vi "Predip.vi"() -> ()   [LabVIEW 2019]
uses:
  <vilib>/NI/Current Value Table/Type Defs/Single Tag.ctl
  <vilib>/NI/Current Value Table/Type Defs/Data Types.ctl
  <vilib>/NI/STM/TCP/Read Meta Data (TCP Ref).vi
  <vilib>/NI/STM/TCP/Get Connection Reference (TCP).vi
  <vilib>/NI/AMC/Read Termination Message.vi
  <vilib>/NI/AMC/Create Single Message.vi
  <vilib>/NI/AMC/Update Message Routing Info.vi
  <vilib>/NI/STM/TCP/Read Meta Data (TCP Clst).vi
  <vilib>/NI/AMC/Globals.vi
  <vilib>/NI/STM/TCP/Write Message (TCP).vi
  <vilib>/NI/AMC/Send Message.vi
  <vilib>/NI/AMC/AMC.lvlib
  <vilib>/NI/STM/NI STM.lvlib
  <vilib>/NI/Current Value Table/Current Value Table.lvlib
panel:
  in  "Sulfuric Proc 1":dbl=2.0 caption="ml Acid Predip" min=0.0 max=2500.0 step=1.0
  in  "Trig Sulfuric Predip":bool caption="Trigger Dose"
  in  "Level Setpoint":dbl(knob)=40.0 min=40.0 max=85.0 step=0.5 scale=40.0..85.0
  in  "Enable Auto Fill":bool
  in  "AcidT3 Flow Last Hr":bool
  in  "AcidT3 Cond Last Hr":bool
  in  "AcidT3 Lev Last Hr":bool
  in  "AcidT3 T Last Hr":bool
  in  "Temperature Setpoint":dbl(knob)=25.0 min=20.0 max=55.0 step=0.5 scale=20.0..55.0
  in  "Enable Heat":bool
  out "Heater 2":bool
  out "Boolean 4":bool
  out "Boolean 2":bool
  out "Boolean 5":bool
  out "Drain":bool
  out "SuckPipe 2":bool
  out "Main Pump":bool
  in  "Tab Control":enum32{"Page 1", "ENG"}(tab)
  out "Heater Enabled":bool
  out "Amps":dbl format="%#.2g"
  out "Volts":dbl format="%#.1f"
  out "VFD T":dbl format="%#.2g"
  out "RPM":dbl format="%#.0f"
  out "Fault Code":dbl format="%#.2g"
  out "Freq":dbl format="%#.2g"
  in  "Drain Predip":bool
  out "Level (L)":dbl(slide) scale=0.0..100.0
  in  "Specific Gravity":dbl(knob)=1.0 min=1.0 max=1.3 step=0.0025 scale=1.0..1.3
  out "E Stop":bool
  out "Run Enabled?":bool
  out "Acid Temperature":dbl(slide) scale=0.0..60.0
  in  "Conductivity":dbl(slide) scale=0.1..1000.0
  in  "Flow Setpoint":dbl(knob)=25.0 min=25.0 max=100.0 step=1.0 scale=25.0..100.0
  in  "Enable Predip":bool
  out "Flow rate":dbl(knob) scale=0.0..100.0
  in  "Machine":bool
  in  "Basement 4":bool
  in  "Dryer":bool
  in  "Rinse 4":bool
  in  "Rinse 3":bool
  in  "Rinse 2":bool
  in  "Basement 3":bool
  in  "Basement 2":bool
  in  "Basement 1":bool
  in  "Plater 6":bool
  in  "Plater 5":bool
  in  "Plater 4":bool
  in  "Plater 3":bool
  in  "Plater 2":bool
  in  "Plater 1":bool
  in  "Predip":bool
  in  "Rinse 1":bool
  in  "Cleaner":bool
  in  "Etch":bool
  out "status":string
  # "Module Selection"
  # "L/min"
  # "mS"
  # "Dosing"
  # "Sulfuric Acid"
  # "Motor Parameters"
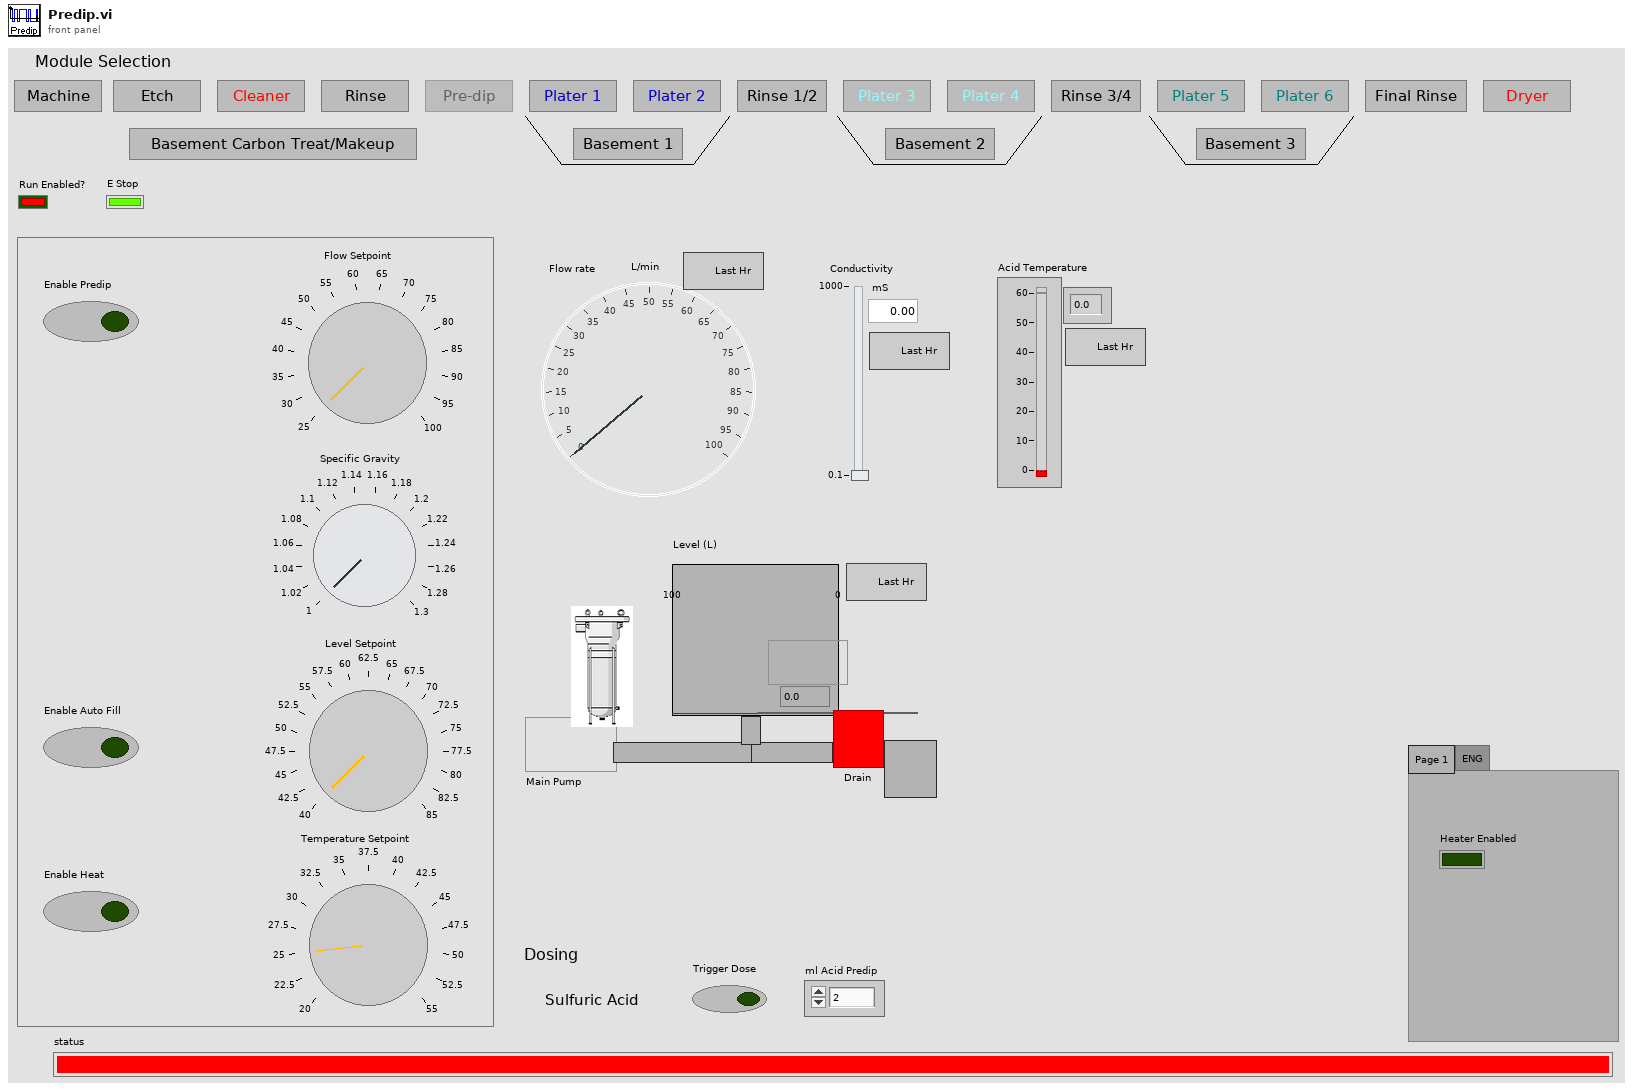
[diagram p1: front panel]
types:
  T1 = typedef "Current Value Table.lvlib/Single Tag.ctl" = cluster{"Data Type":T2, "Name":string, "Value":string, "Description":string}
  T2 = typedef "Current Value Table.lvlib/Data Types.ctl" = enum16{"Double", "Single", "I64", "I32", "I16", "I8", "U64", "U32", "U16", "U8", "String", "Boolean", "Array of U8", "Array of U16", "Array of U32", "Array of U64", "Array of I64", "Array of I32", "Array of I16", "Array of I8", "Array of Double", "Array of Single", "Array of Boolean", "Array of String"}
  T3 = typedef "NI STM.lvlib/TCP Connection Info.ctl" = cluster{"connection ID":refnum<k5>, "meta data":T4[]}
  T4 = typedef "NI STM.lvlib/MetaDataElement.ctl" = string
  T5 = typedef "AMC.lvlib/Message Queue.ctl" = refnum<queue>
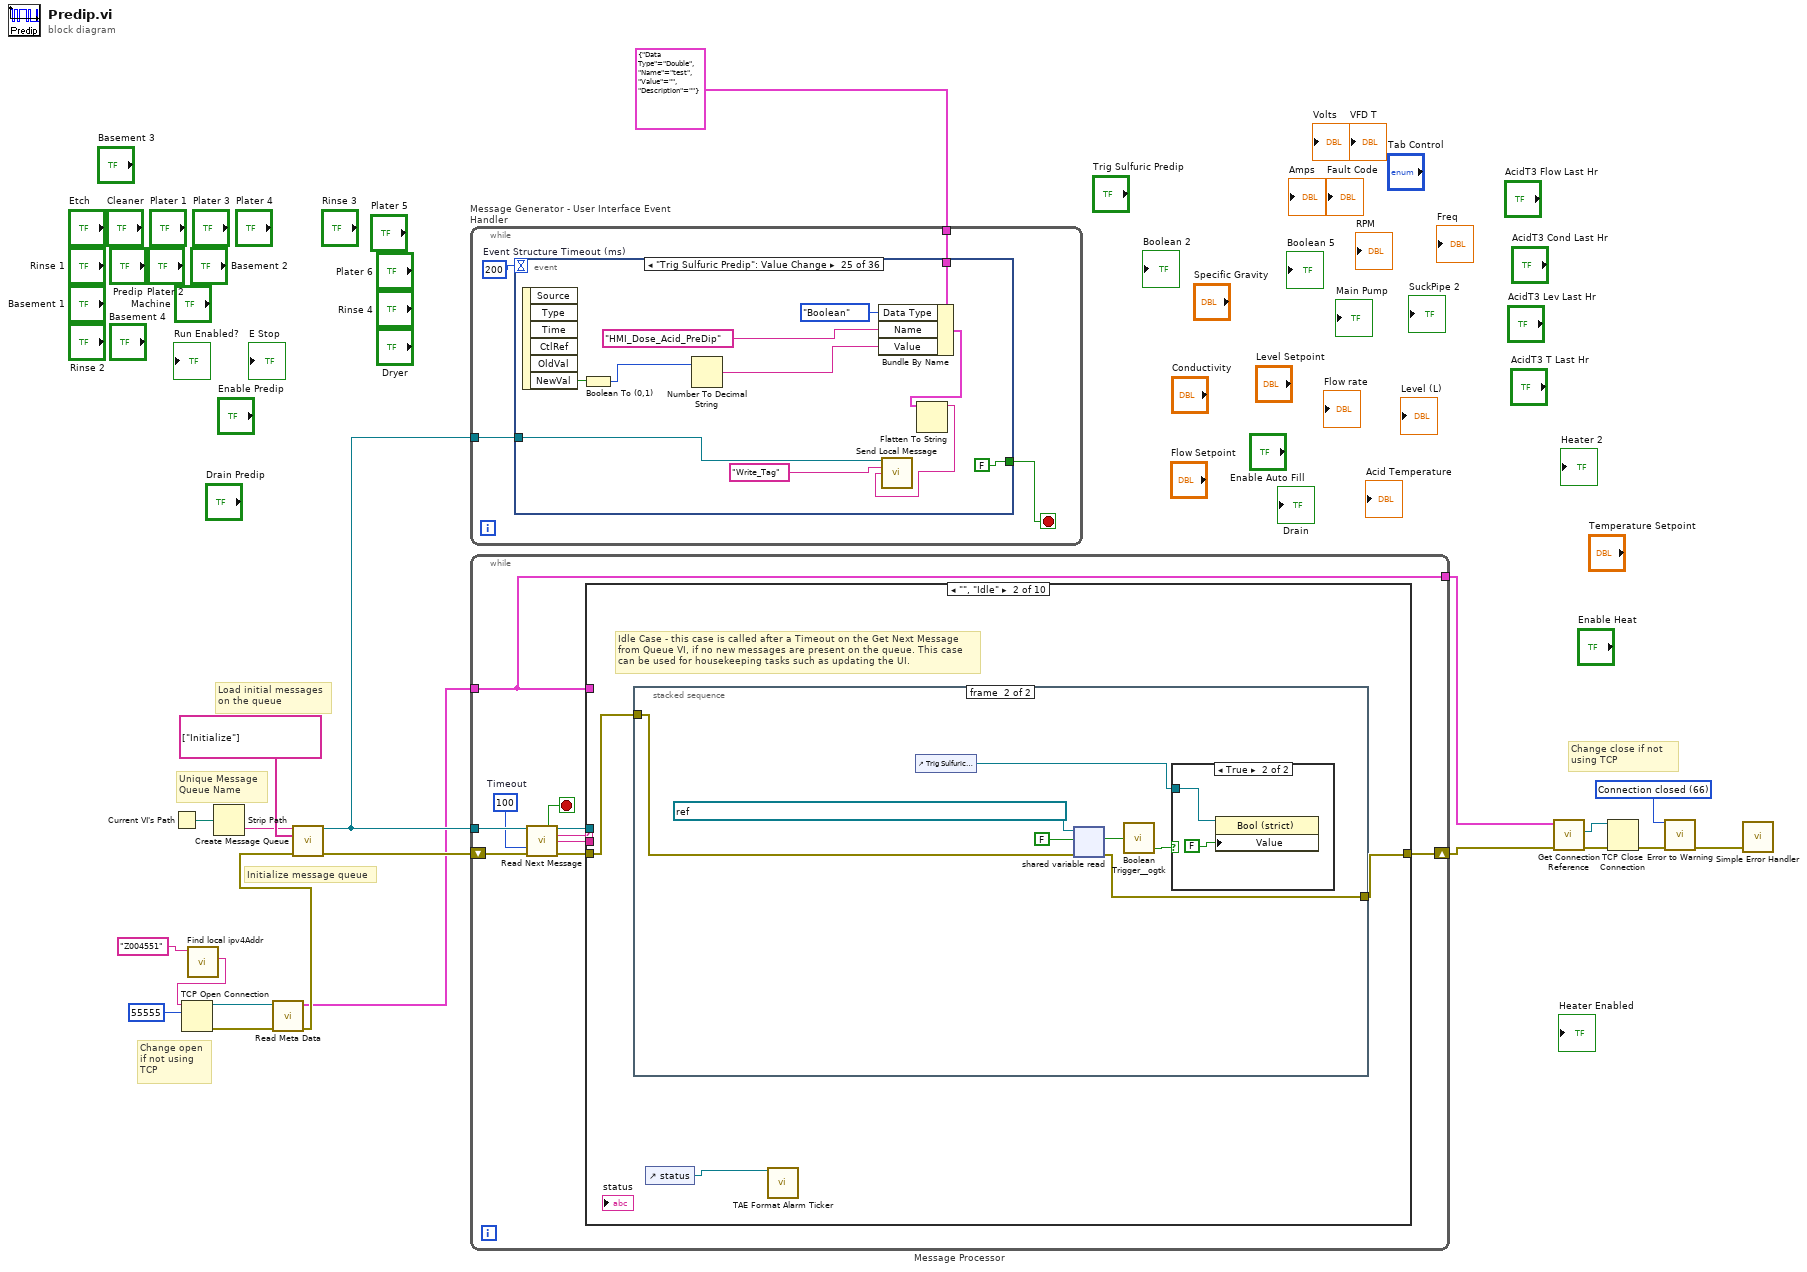
[diagram p0: block diagram]
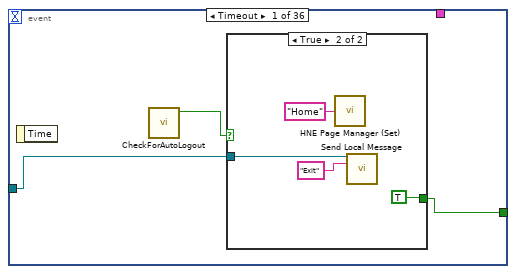
[diagram p2: hidden frame]
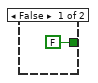
[diagram p3: hidden frame]
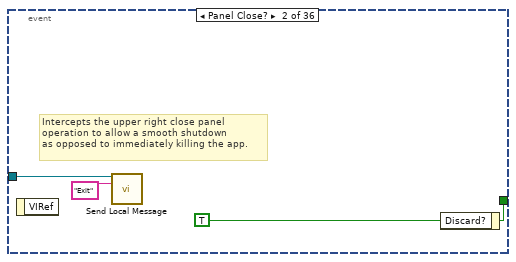
[diagram p4: hidden frame]
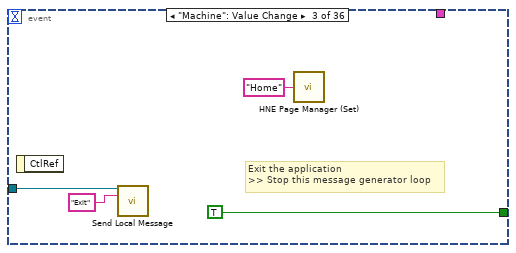
[diagram p5: hidden frame]
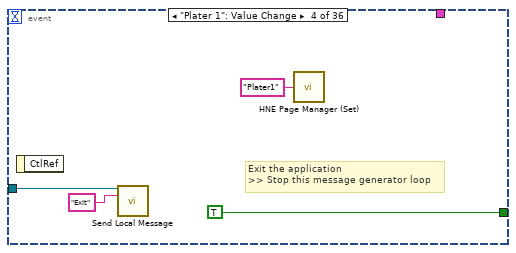
[diagram p6: hidden frame]
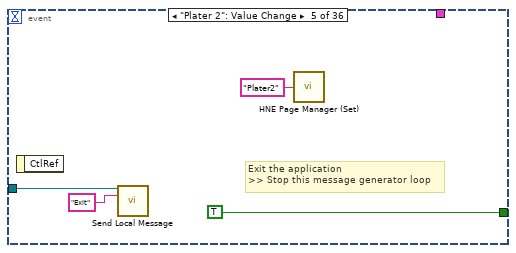
[diagram p7: hidden frame]
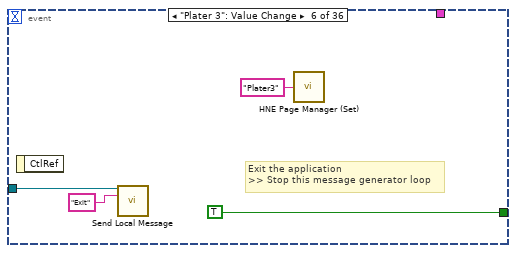
[diagram p8: hidden frame]
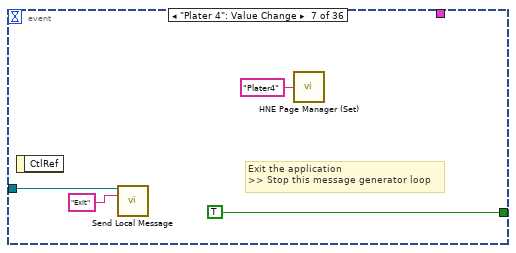
[diagram p9: hidden frame]
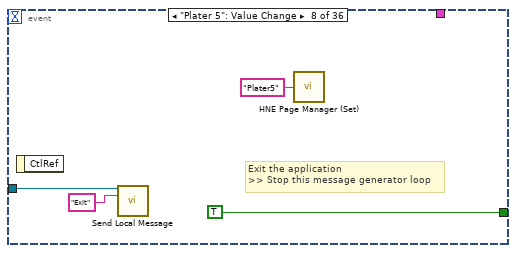
[diagram p10: hidden frame]
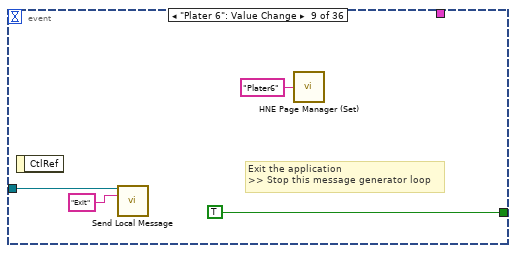
[diagram p11: hidden frame]
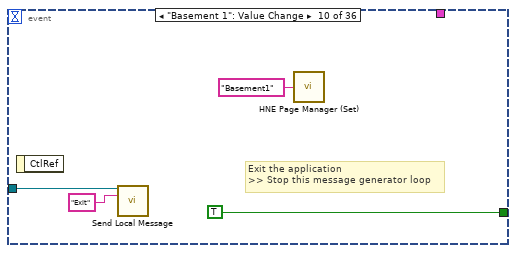
[diagram p12: hidden frame]
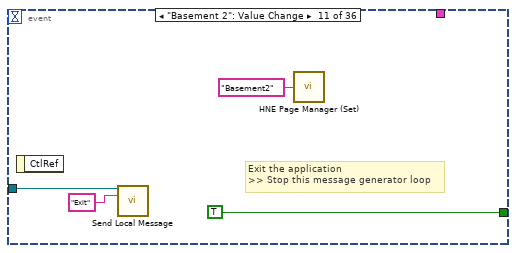
[diagram p13: hidden frame]
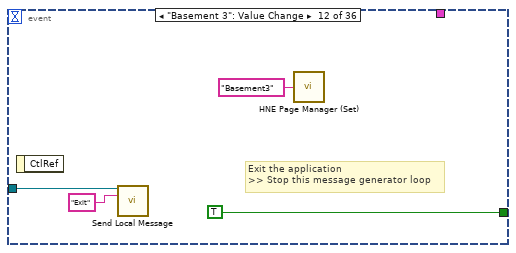
[diagram p14: hidden frame]
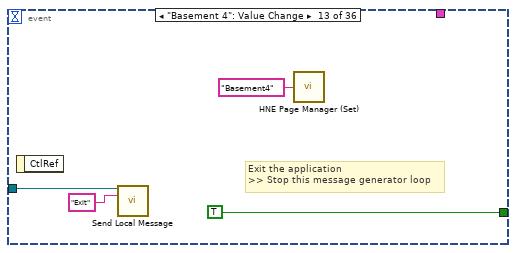
[diagram p15: hidden frame]
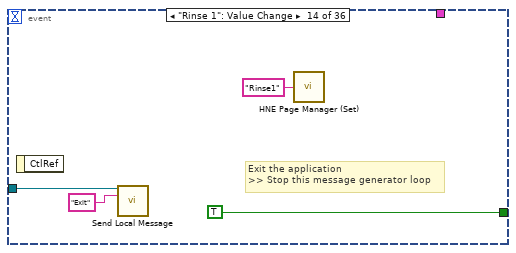
[diagram p16: hidden frame]
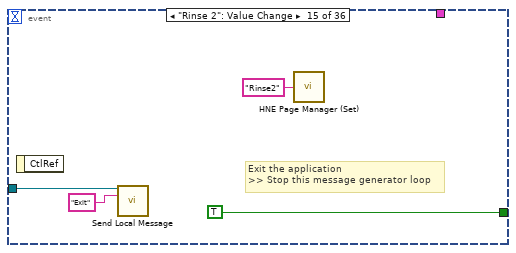
[diagram p17: hidden frame]
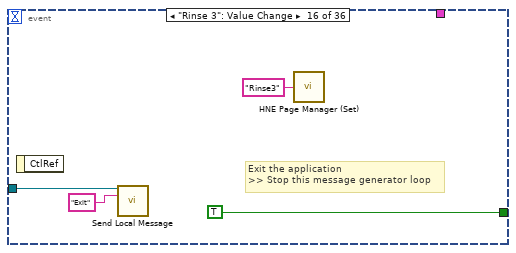
[diagram p18: hidden frame]
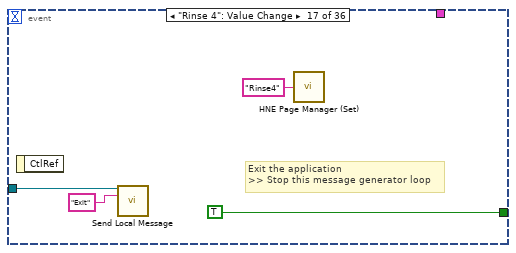
[diagram p19: hidden frame]
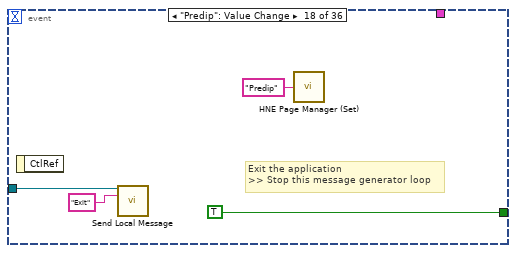
[diagram p20: hidden frame]
diagram:
  w9 = 66 items=["No Error", "Argument Error", "Memory Full", "Out of Zone", "End of File", "File Already Open", "Generic File IO Error", "File Not Found", "File Permission Error", "Disk Full", "Duplicate Path", "Too Many Files Open", "Not Enabled", "Resource File Not Found", "Cannot Add Resource", "Resource Not Found", "Image Not Found", "Image Memory Error", "Pen Does Not Exist", "Config Bad Type", "Config Token Not Found", "Config Parse Error", "Config Memory Error", "Bad External Code Format", "Bad External Code Offset", "External Code Not Present", "Null Window", "Destroy Window Mixup", "Null Menu", "Print Aborted", "Bad Print Record", "Print Driver Error", "Windows Error During Print", "Memory Error During Print", "Print Dialog Error", "Generic Print Error", "Invalid Device Refnum", "Device Not Found", "Device Parameter Error", "Device Unit Error", "Can't Open Device", "Device Call Aborted", "Generic Error", "Cancelled By User", "Object ID Too Low", "Object ID Too High", "Object Not In Heap", "Unknown Heap", "Bad DefProc ID", "DefProc Not In Table", "Message Out Of Range", "Null Method", "Unknown Message", "Manager Call Not Supported", "Bad address", "Connection In progress", "Connection timed out", "Connection is already in progress", "Network attribute not supported", "Network error", "Address in use", "System out of memory", "Connection aborted", "Connection refused", "Connection is not connected", "Connection is already connected", "Connection closed", "Initialize error (interapplication manager)", "Bad occurrence", "Wait on unbound occurrence handler", "Occurrence queue overflow", "Bad path", "Semaphore not signaled", "Unrecognized type (interapplication manager)"] ("1st Error to Convert")
  # "Change close if not using TCP"
  # "Change open if not using TCP"
  # "Initialize message queue"
  # "Unique Message\nQueue Name"
  # "Load initial messages\non the queue"
  n1 = Current VI's Path() -> (path=w16:path)
  n2 = call "Find local ipv4Addr.vi"("MachineToFind"="Z004551" ("Target IP Address")) -> ("name"=w2:string)  [unwired: 9 in, 1 out]
  n3 = TCP Open Connection(address=w2, remote port or service name=u16 55555 ("remote port")) -> (connection ID=w14:refnum<k5>, error out=w13:errorcluster)  [unwired: 1 in, 2 out]
  n4 = Strip Path(path=w16) -> (name=w19:string)  [unwired: 1 out]
  n5 = call-poly <vilib>:"Read Meta Data.vi"("error in"=w13, "connection ID"=w14) -> ("error out"=w12:errorcluster, "connection info out"=w11:T3)  [unwired: 7 in, 1 out]
  n6 = call <vilib>:"Create Message Queue.vi"("message queue name"=w19, "initial message names"=string[] ["Initialize"], "error in"=w12) -> ("message queue out"=w18:T5, "error out"=w17:errorcluster)  [unwired: 11 in]
  n7 = while "Message Generator - User Interface Event Handler" {
    tunnel: w18 -> [w22]
    tunnel: T1 {"Data Type"=enum."Double", "Name"="test", "Value"="", "Description"=""} ("Tag") -> [w21]
    stop <- w23 stop-if-true
    w24 = 200  # Event Structure Timeout (ms)
    n8 = event shown="[24] \"Trig Sulfuric Predip\": Value Change" {
      selector: _ -> [_ _ _ _ _ _ _ _ _ _ _ _ _ _ _ _ _ _ _ _ _ _ _ _ _ _ _ _ _ _ _ _ _ _ _ _]
      dyn-events: _ -> [_ _ _ _ _ _ _ _ _ _ _ _ _ _ _ _ _ _ _ _ _ _ _ _ _ _ _ _ _ _ _ _ _ _ _ _]
      timeout: w24 -> [_ _ _ _ _ _ _ _ _ _ _ _ _ _ _ _ _ _ _ _ _ _ _ _ _ _ _ _ _ _ _ _ _ _ _ _]
      tunnel: [w25 w35 TRUE ("Discard?") TRUE ("Discard?") TRUE ("Discard?") TRUE ("Discard?") TRUE ("Discard?") TRUE ("Discard?") TRUE ("Discard?") TRUE ("Discard?") TRUE ("Discard?") TRUE ("Discard?") TRUE ("Discard?") TRUE ("Discard?") TRUE ("Discard?") TRUE ("Discard?") TRUE ("Discard?") TRUE ("Discard?") TRUE ("Discard?") TRUE ("Discard?") TRUE ("Discard?") FALSE ("Discard?") FALSE ("Discard?") FALSE ("Discard?") FALSE ("Discard?") _ _ _ _ FALSE ("Discard?") FALSE ("Discard?") FALSE ("Discard?") FALSE ("Discard?") FALSE ("Discard?") FALSE ("Discard?") _] -> w23
      tunnel: w22 -> [w26 w33 w37 w41 w45 w49 w53 w57 w61 w65 w69 w73 w77 w81 w85 w89 w93 w97 w101 w105 w109 w120 w131 w142 w153 w156 w161 w166 w171 w179 w190 w200 w210 w220 w230 w233]
      tunnel: w21 -> [_ _ _ _ _ _ _ _ _ _ _ _ _ _ _ _ _ _ _ _ _ w114 w125 w136 w147 _ _ _ _ _ w186 w196 w206 w216 w226 _]
      event Timeout {
        n9 = event-data() -> ()  [unwired: 2 out]
        n10 = call "CheckForAutoLogout.vi"() -> ("Boolean"=w27:bool)  [unwired: 11 in]
        n11 = case shown="True" w27 {
          tunnel: [FALSE ("Discard?") TRUE ("Discard?")] -> w25
          tunnel: w26 -> [_ w29]
          frame False {
          }
          frame True {
            n12 = call <userlib>:"HNE Page Manager (Set).vi"("Next Page"="Home") -> ()  [unwired: 4 in, 1 out]
            n13 = call <vilib>:"Send Local Message.vi"("message queue in"=w29, "message name"="Exit") -> ()  [unwired: 11 in, 3 out]
          }
        }
      }
      event Panel Close? {
        w35 = TRUE ("Discard?")
        # "Intercepts the upper right close panel\noperation to allow a smooth shutdown\nas opposed to immediately killing the app."
        n14 = event-data() -> ()  [unwired: 2 out]
        n15 = call <vilib>:"Send Local Message.vi"("message queue in"=w33, "message name"="Exit") -> ()  [unwired: 11 in, 3 out]
        n16 = event-data("Discard?"=w35) -> ()  [unwired: 1 in, 1 out]
      }
      event "Machine": Value Change {
        # "Exit the application\n>> Stop this message generator loop"
        n17 = event-data() -> ()  [unwired: 2 out]
        n18 = call <vilib>:"Send Local Message.vi"("message queue in"=w37, "message name"="Exit") -> ()  [unwired: 11 in, 3 out]
        n19 = call <userlib>:"HNE Page Manager (Set).vi"("Next Page"="Home") -> ()  [unwired: 4 in, 1 out]
      }
      event "Plater 1": Value Change {
        # "Exit the application\n>> Stop this message generator loop"
        n20 = event-data() -> ()  [unwired: 2 out]
        n21 = call <vilib>:"Send Local Message.vi"("message queue in"=w41, "message name"="Exit") -> ()  [unwired: 11 in, 3 out]
        n22 = call <userlib>:"HNE Page Manager (Set).vi"("Next Page"="Plater1") -> ()  [unwired: 4 in, 1 out]
      }
      event "Plater 2": Value Change {
        # "Exit the application\n>> Stop this message generator loop"
        n23 = event-data() -> ()  [unwired: 2 out]
        n24 = call <vilib>:"Send Local Message.vi"("message queue in"=w45, "message name"="Exit") -> ()  [unwired: 11 in, 3 out]
        n25 = call <userlib>:"HNE Page Manager (Set).vi"("Next Page"="Plater2") -> ()  [unwired: 4 in, 1 out]
      }
      event "Plater 3": Value Change {
        # "Exit the application\n>> Stop this message generator loop"
        n26 = event-data() -> ()  [unwired: 2 out]
        n27 = call <vilib>:"Send Local Message.vi"("message queue in"=w49, "message name"="Exit") -> ()  [unwired: 11 in, 3 out]
        n28 = call <userlib>:"HNE Page Manager (Set).vi"("Next Page"="Plater3") -> ()  [unwired: 4 in, 1 out]
      }
      event "Plater 4": Value Change {
        # "Exit the application\n>> Stop this message generator loop"
        n29 = event-data() -> ()  [unwired: 2 out]
        n30 = call <vilib>:"Send Local Message.vi"("message queue in"=w53, "message name"="Exit") -> ()  [unwired: 11 in, 3 out]
        n31 = call <userlib>:"HNE Page Manager (Set).vi"("Next Page"="Plater4") -> ()  [unwired: 4 in, 1 out]
      }
      event "Plater 5": Value Change {
        # "Exit the application\n>> Stop this message generator loop"
        n32 = event-data() -> ()  [unwired: 2 out]
        n33 = call <vilib>:"Send Local Message.vi"("message queue in"=w57, "message name"="Exit") -> ()  [unwired: 11 in, 3 out]
        n34 = call <userlib>:"HNE Page Manager (Set).vi"("Next Page"="Plater5") -> ()  [unwired: 4 in, 1 out]
      }
      event "Plater 6": Value Change {
        # "Exit the application\n>> Stop this message generator loop"
        n35 = event-data() -> ()  [unwired: 2 out]
        n36 = call <vilib>:"Send Local Message.vi"("message queue in"=w61, "message name"="Exit") -> ()  [unwired: 11 in, 3 out]
        n37 = call <userlib>:"HNE Page Manager (Set).vi"("Next Page"="Plater6") -> ()  [unwired: 4 in, 1 out]
      }
      event "Basement 1": Value Change {
        # "Exit the application\n>> Stop this message generator loop"
        n38 = event-data() -> ()  [unwired: 2 out]
        n39 = call <vilib>:"Send Local Message.vi"("message queue in"=w65, "message name"="Exit") -> ()  [unwired: 11 in, 3 out]
        n40 = call <userlib>:"HNE Page Manager (Set).vi"("Next Page"="Basement1") -> ()  [unwired: 4 in, 1 out]
      }
      event "Basement 2": Value Change {
        # "Exit the application\n>> Stop this message generator loop"
        n41 = event-data() -> ()  [unwired: 2 out]
        n42 = call <vilib>:"Send Local Message.vi"("message queue in"=w69, "message name"="Exit") -> ()  [unwired: 11 in, 3 out]
        n43 = call <userlib>:"HNE Page Manager (Set).vi"("Next Page"="Basement2") -> ()  [unwired: 4 in, 1 out]
      }
      event "Basement 3": Value Change {
        # "Exit the application\n>> Stop this message generator loop"
        n44 = event-data() -> ()  [unwired: 2 out]
        n45 = call <vilib>:"Send Local Message.vi"("message queue in"=w73, "message name"="Exit") -> ()  [unwired: 11 in, 3 out]
        n46 = call <userlib>:"HNE Page Manager (Set).vi"("Next Page"="Basement3") -> ()  [unwired: 4 in, 1 out]
      }
      event "Basement 4": Value Change {
        # "Exit the application\n>> Stop this message generator loop"
        n47 = event-data() -> ()  [unwired: 2 out]
        n48 = call <vilib>:"Send Local Message.vi"("message queue in"=w77, "message name"="Exit") -> ()  [unwired: 11 in, 3 out]
        n49 = call <userlib>:"HNE Page Manager (Set).vi"("Next Page"="Basement4") -> ()  [unwired: 4 in, 1 out]
      }
      event "Rinse 1": Value Change {
        # "Exit the application\n>> Stop this message generator loop"
        n50 = event-data() -> ()  [unwired: 2 out]
        n51 = call <vilib>:"Send Local Message.vi"("message queue in"=w81, "message name"="Exit") -> ()  [unwired: 11 in, 3 out]
        n52 = call <userlib>:"HNE Page Manager (Set).vi"("Next Page"="Rinse1") -> ()  [unwired: 4 in, 1 out]
      }
      event "Rinse 2": Value Change {
        # "Exit the application\n>> Stop this message generator loop"
        n53 = event-data() -> ()  [unwired: 2 out]
        n54 = call <vilib>:"Send Local Message.vi"("message queue in"=w85, "message name"="Exit") -> ()  [unwired: 11 in, 3 out]
        n55 = call <userlib>:"HNE Page Manager (Set).vi"("Next Page"="Rinse2") -> ()  [unwired: 4 in, 1 out]
      }
      event "Rinse 3": Value Change {
        # "Exit the application\n>> Stop this message generator loop"
        n56 = event-data() -> ()  [unwired: 2 out]
        n57 = call <vilib>:"Send Local Message.vi"("message queue in"=w89, "message name"="Exit") -> ()  [unwired: 11 in, 3 out]
        n58 = call <userlib>:"HNE Page Manager (Set).vi"("Next Page"="Rinse3") -> ()  [unwired: 4 in, 1 out]
      }
      event "Rinse 4": Value Change {
        # "Exit the application\n>> Stop this message generator loop"
        n59 = event-data() -> ()  [unwired: 2 out]
        n60 = call <vilib>:"Send Local Message.vi"("message queue in"=w93, "message name"="Exit") -> ()  [unwired: 11 in, 3 out]
        n61 = call <userlib>:"HNE Page Manager (Set).vi"("Next Page"="Rinse4") -> ()  [unwired: 4 in, 1 out]
      }
      event "Predip": Value Change {
        # "Exit the application\n>> Stop this message generator loop"
        n62 = event-data() -> ()  [unwired: 2 out]
        n63 = call <vilib>:"Send Local Message.vi"("message queue in"=w97, "message name"="Exit") -> ()  [unwired: 11 in, 3 out]
        n64 = call <userlib>:"HNE Page Manager (Set).vi"("Next Page"="Predip") -> ()  [unwired: 4 in, 1 out]
      }
      event "Cleaner": Value Change {
        # "Exit the application\n>> Stop this message generator loop"
        n65 = event-data() -> ()  [unwired: 2 out]
        n66 = call <vilib>:"Send Local Message.vi"("message queue in"=w101, "message name"="Exit") -> ()  [unwired: 11 in, 3 out]
        n67 = call <userlib>:"HNE Page Manager (Set).vi"("Next Page"="Clean") -> ()  [unwired: 4 in, 1 out]
      }
      event "Etch": Value Change {
        # "Exit the application\n>> Stop this message generator loop"
        n68 = event-data() -> ()  [unwired: 2 out]
        n69 = call <vilib>:"Send Local Message.vi"("message queue in"=w105, "message name"="Exit") -> ()  [unwired: 11 in, 3 out]
        n70 = call <userlib>:"HNE Page Manager (Set).vi"("Next Page"="Etch") -> ()  [unwired: 4 in, 1 out]
      }
      event "Dryer": Value Change {
        # "Exit the application\n>> Stop this message generator loop"
        n71 = event-data() -> ()  [unwired: 2 out]
        n72 = call <vilib>:"Send Local Message.vi"("message queue in"=w109, "message name"="Exit") -> ()  [unwired: 11 in, 3 out]
        n73 = call <userlib>:"HNE Page Manager (Set).vi"("Next Page"="Dryer") -> ()  [unwired: 4 in, 1 out]
      }
      event "Enable Predip": Value Change {
        n74 = event-data() -> ("NewVal"=w119:bool)  [unwired: 6 out]
        n75 = Boolean To (0,1)(Boolean=w119) -> (0, 1=w118:i16)
        n76 = Number To Decimal String(number=w118) -> (decimal integer string=w113:string)  [unwired: 1 in]
        n77 = Bundle By Name(cluster=w114, "Data Type"=Data_Types."Boolean", "Name"="HMI_ATank3_Enable", "Value"=w113) -> (w115:T1)
        n78 = Flatten To String(anything=w115) -> (data string=w112:string)  [unwired: 3 in, 2 out]
        n79 = call <vilib>:"Send Local Message.vi"("message queue in"=w120, "message name"="Write_Tag", "message value"=w112) -> ()  [unwired: 10 in, 3 out]
      }
      event "Enable Heat": Value Change {
        n80 = event-data() -> ("NewVal"=w130:bool)  [unwired: 6 out]
        n81 = Boolean To (0,1)(Boolean=w130) -> (0, 1=w129:i16)
        n82 = Number To Decimal String(number=w129) -> (decimal integer string=w124:string)  [unwired: 1 in]
        n83 = Bundle By Name(cluster=w125, "Data Type"=Data_Types."Boolean", "Name"="HMI_ATank3_HeatEnable", "Value"=w124) -> (w126:T1)
        n84 = Flatten To String(anything=w126) -> (data string=w123:string)  [unwired: 3 in, 2 out]
        n85 = call <vilib>:"Send Local Message.vi"("message queue in"=w131, "message name"="Write_Tag", "message value"=w123) -> ()  [unwired: 10 in, 3 out]
      }
      event "Enable Auto Fill": Value Change {
        n86 = event-data() -> ("NewVal"=w141:bool)  [unwired: 6 out]
        n87 = Boolean To (0,1)(Boolean=w141) -> (0, 1=w140:i16)
        n88 = Number To Decimal String(number=w140) -> (decimal integer string=w135:string)  [unwired: 1 in]
        n89 = Bundle By Name(cluster=w136, "Data Type"=Data_Types."Boolean", "Name"="HMI_ATank3_Fill_To_Level", "Value"=w135) -> (w137:T1)
        n90 = Flatten To String(anything=w137) -> (data string=w134:string)  [unwired: 3 in, 2 out]
        n91 = call <vilib>:"Send Local Message.vi"("message queue in"=w142, "message name"="Write_Tag", "message value"=w134) -> ()  [unwired: 10 in, 3 out]
      }
      event "Trig Sulfuric Predip": Value Change {
        n92 = event-data() -> ("NewVal"=w152:bool)  [unwired: 6 out]
        n93 = Boolean To (0,1)(Boolean=w152) -> (0, 1=w151:i16)
        n94 = Number To Decimal String(number=w151) -> (decimal integer string=w146:string)  [unwired: 1 in]
        n95 = Bundle By Name(cluster=w147, "Data Type"=Data_Types."Boolean", "Name"="HMI_Dose_Acid_PreDip", "Value"=w146) -> (w148:T1)
        n96 = Flatten To String(anything=w148) -> (data string=w145:string)  [unwired: 3 in, 2 out]
        n97 = call <vilib>:"Send Local Message.vi"("message queue in"=w153, "message name"="Write_Tag", "message value"=w145) -> ()  [unwired: 10 in, 3 out]
      }
      event "AcidT3 T Last Hr": Value Change {
        n98 = event-data() -> ("NewVal"=w157:bool)  [unwired: 6 out]
        n99 = case shown="True" w157 {
          tunnel: w156 -> [_ w160]
          frame False {
          }
          frame True {
            n100 = call <vilib>:"Send Local Message.vi"("message queue in"=w160, "message name"="DisplayLastHr", "message value"="Acid3_Temperature") -> ()  [unwired: 10 in, 3 out]
          }
        }
      }
      event "AcidT3 Lev Last Hr": Value Change {
        n101 = event-data() -> ("NewVal"=w162:bool)  [unwired: 6 out]
        n102 = case shown="True" w162 {
          tunnel: w161 -> [_ w165]
          frame False {
          }
          frame True {
            n103 = call <vilib>:"Send Local Message.vi"("message queue in"=w165, "message name"="DisplayLastHr", "message value"="Acid3_Level") -> ()  [unwired: 10 in, 3 out]
          }
        }
      }
      event "AcidT3 Cond Last Hr": Value Change {
        n104 = event-data() -> ("NewVal"=w167:bool)  [unwired: 6 out]
        n105 = case shown="True" w167 {
          tunnel: w166 -> [_ w170]
          frame False {
          }
          frame True {
            n106 = call <vilib>:"Send Local Message.vi"("message queue in"=w170, "message name"="DisplayLastHr", "message value"="Acid3_Conductivity") -> ()  [unwired: 10 in, 3 out]
          }
        }
      }
      event "AcidT3 Flow Last Hr": Value Change {
        n107 = event-data() -> ("NewVal"=w172:bool)  [unwired: 6 out]
        n108 = case shown="True" w172 {
          tunnel: w171 -> [_ w175]
          frame False {
          }
          frame True {
            n109 = call <vilib>:"Send Local Message.vi"("message queue in"=w175, "message name"="DisplayLastHr", "message value"="Acid3_Flow") -> ()  [unwired: 10 in, 3 out]
          }
        }
      }
      event "Drain Predip", "Drain": Value Change {
        n110 = event-data() -> ("NewVal"=w177:bool)  [unwired: 6 out]
        n111 = case shown="True" w177 {
          tunnel: [FALSE ("Drain?") w182] -> w176
          frame False {
          }
          frame True {
            # "Verify drain"
            n112 = call "Drain to AMB verify dialog.vi"() -> ("Drain?"=w182:bool)  [unwired: 11 in]
          }
        }
        n113 = call "Write Boolean To Que.vi"("Tag"="HMI_ATank3_Drain", "NewVal"=w176, "Queue in"=w179) -> ()  [unwired: 9 in]
        n114 = local write "Drain Predip"(w176) -> ()
        n115 = local write "Drain"(w176) -> ()
      }
      event "Flow Setpoint": Value Change {
        n116 = event-data() -> ("NewVal"=w184:dbl)  [unwired: 6 out]
        n117 = Number To Fractional String(number=w184) -> (F-format string=w183:string)  [unwired: 3 in]
        n118 = Bundle By Name(cluster=w186, "Data Type"=Data_Types."Double", "Name"="HMI_ATNK3_Flow_Setpoint", "Value"=w183) -> (w187:T1)
        n119 = Flatten To String(anything=w187) -> (data string=w185:string)  [unwired: 3 in, 2 out]
        n120 = call <vilib>:"Send Local Message.vi"("message queue in"=w190, "message name"="Write_Tag", "message value"=w185) -> ()  [unwired: 10 in, 3 out]
      }
      event "Specific Gravity": Value Change {
        n121 = event-data() -> ("NewVal"=w194:dbl)  [unwired: 6 out]
        n122 = Number To Fractional String(number=w194) -> (F-format string=w193:string)  [unwired: 3 in]
        n123 = Bundle By Name(cluster=w196, "Data Type"=Data_Types."Double", "Name"="HMI_Acid3_Tank_SG", "Value"=w193) -> (w197:T1)
        n124 = Flatten To String(anything=w197) -> (data string=w195:string)  [unwired: 3 in, 2 out]
        n125 = call <vilib>:"Send Local Message.vi"("message queue in"=w200, "message name"="Write_Tag", "message value"=w195) -> ()  [unwired: 10 in, 3 out]
      }
      event "Temperature Setpoint": Value Change {
        n126 = event-data() -> ("NewVal"=w204:dbl)  [unwired: 6 out]
        n127 = Number To Fractional String(number=w204) -> (F-format string=w203:string)  [unwired: 3 in]
        n128 = Bundle By Name(cluster=w206, "Data Type"=Data_Types."Double", "Name"="HMI_ATNK3_T_Setpoint", "Value"=w203) -> (w207:T1)
        n129 = Flatten To String(anything=w207) -> (data string=w205:string)  [unwired: 3 in, 2 out]
        n130 = call <vilib>:"Send Local Message.vi"("message queue in"=w210, "message name"="Write_Tag", "message value"=w205) -> ()  [unwired: 10 in, 3 out]
      }
      event "Level Setpoint": Value Change {
        n131 = event-data() -> ("NewVal"=w214:dbl)  [unwired: 6 out]
        n132 = Number To Fractional String(number=w214) -> (F-format string=w213:string)  [unwired: 3 in]
        n133 = Bundle By Name(cluster=w216, "Data Type"=Data_Types."Double", "Name"="HMI_ATank3_Level_SetPnt", "Value"=w213) -> (w217:T1)
        n134 = Flatten To String(anything=w217) -> (data string=w215:string)  [unwired: 3 in, 2 out]
        n135 = call <vilib>:"Send Local Message.vi"("message queue in"=w220, "message name"="Write_Tag", "message value"=w215) -> ()  [unwired: 10 in, 3 out]
      }
      event "Sulfuric Proc 1": Value Change {
        n136 = event-data() -> ("NewVal"=w224:dbl)  [unwired: 6 out]
        n137 = Number To Fractional String(number=w224) -> (F-format string=w223:string)  [unwired: 3 in]
        n138 = Bundle By Name(cluster=w226, "Data Type"=Data_Types."Double", "Name"="HMI_Acid_Amount_PreDip", "Value"=w223) -> (w227:T1)
        n139 = Flatten To String(anything=w227) -> (data string=w225:string)  [unwired: 3 in, 2 out]
        n140 = call <vilib>:"Send Local Message.vi"("message queue in"=w230, "message name"="Write_Tag", "message value"=w225) -> ()  [unwired: 10 in, 3 out]
      }
      event Menu Selection (User) {
        # "Add run-time menu items to the message\nqueue. The message handler case names must match the menu ItemTag names."
        n141 = event-data() -> ("ItemTag"=w234:string)  [unwired: 1 out]
        n142 = call <vilib>:"Send Local Message.vi"("message queue in"=w233, "message name"=w234) -> ()  [unwired: 11 in, 3 out]
      }
    }
  }
  n143 = while "Message Processor" {
    shift-left: w17 -> [w240]
    shift-right: [w244] -> w4
    tunnel: w18 -> [w241]
    tunnel: w11 -> [w235]
    tunnel: [w235] -> w5
    stop <- w243 stop-if-true
    w236 = 100  # Timeout
    n144 = call <vilib>:"Read Next Message.vi"("message queue in"=w241, "timeout (1 ms)"=w236, "error in"=w240) -> ("exit process?"=w243:bool, "message queue out"=w242:T5, "message name"=w238:string, "message value"=w237:string, "error out"=w239:errorcluster)  [unwired: 5 in, 3 out]
    n145 = case shown="\"\", \"Idle\"" w238 {
      selector: w238 -> [_ _ w263 _ _ _ _ _ _ _]
      tunnel: w242 -> [_ _ _ _ _ _ w301 _ _ _]
      tunnel: w239 -> [w245 w247 w264 w265 w267 w285 w302 w304 w308 w310]
      tunnel: [w245 w246 w264 errorcluster {"status"=FALSE, "code"=0, "source"=""} ("error out") w267 w284 w300 w304 w307 w310] -> w244
      tunnel: w237 -> [_ _ _ _ _ _ _ _ w305 w311]
      tunnel: w235 -> [_ _ _ _ _ _ _ _ w306 _]
      frame "---------- Framework Operations ----------" {
        # "Dummy case to add a seperator in the Case Structure menu"
      }
      frame "", "Idle" {
        # "Idle Case - this case is called after a Timeout on the Get Next Message from Queue VI, if no new messages are present on the queue. This case can be used for housekeeping tasks such as updating the UI."
        n146 = stacked-sequence {
          tunnel: w247 -> [_ w253]
          tunnel: [_ w252] -> w246
          frame #0 {
            n147 = local read "Main Pump"() -> (w250:bool)
            n148 = local read "Drain"() -> (w249:bool)
            n149 = Or(x=w249, y=w250) -> (x .or. y?=→"Boolean 4":bool)
          }
          frame #1 {
            n150 = control-ref of="Trig Sulfuric Predip"() -> (w254:refnum<vi>)
            n151 = shared-variable-read(refnum<k21> "ni.var.psp://z004551/CDL0100 ReadWriteTags/HMI_Dose_Acid_PreDip" ("shared variable refnum in"), w253, FALSE) -> (w252:errorcluster, w256:bool)  [unwired: 2 out]
            n152 = call <userlib>:"Boolean Trigger__ogtk.vi"("Boolean Input"=w256) -> ("Falling Edge"=w255:bool)  [unwired: 1 in, 1 out]
            n153 = case shown="True" w255 {
              tunnel: w254 -> [_ w260]
              frame False {
              }
              frame True {
                n154 = property class="Bool (strict)"(reference=w260, "Value"=FALSE) -> ()  [unwired: 1 in, 2 out]
              }
            }
          }
        }
        n155 = control-ref of="status"() -> (w248:refnum<vi>)
        n156 = call <userlib>:"TAE Format Alarm Ticker.vi"("Alarm Ticker Ref"=w248) -> ()  [unwired: 15 in]
      }
      frame "Missing Message Handler", Default {
        # "Call this case if a message is received that is not handled \nby any other case. Typically this is a programming error\nas a result of a typo or unhandled message/missing message handler."
        n157 = Format Into String(format string="DevError: Missing message handler for '%s\" message." ("message"), w263) -> (resulting string=w261:string)  [unwired: 2 in, 1 out]
        n158 = One Button Dialog(message=w261) -> ()  [unwired: 2 out]
      }
      frame "Error" {
        # "General Error Case - this case is called if an error is passed using the error cluster below. Typically most new errors should be handed in each individual case and not passed in the rror cluster. If necessary a custom error handler case should be added and called from other cases."
        n159 = call <vilib>:"Simple Error Handler.vi"("error in (no error)"=w265) -> ()  [unwired: 1 in, 8 out]
      }
      frame "---------- Generic Operations ----------" {
        # "Dummy case to add a seperator in the Case Structure menu"
      }
      frame "Initialize" {
        # "Initialize the state variables and user interface"
        n160 = shared-variable-read(refnum<k21> "ni.var.psp://z004551/CDL0100 ReadWriteTags/HMI_ATank3_Drain" ("shared variable refnum in"), FALSE) -> (w288:bool)  [unwired: 1 in, 3 out]
        n161 = shared-variable-read(refnum<k21> "ni.var.psp://z004551/CDL0100 ReadWriteTags/HMI_ATank3_Enable" ("shared variable refnum in"), FALSE) -> (w297:bool)  [unwired: 1 in, 3 out]
        n162 = shared-variable-read(refnum<k21> "ni.var.psp://z004551/CDL0100 ReadWriteTags/HMI_ATank3_Fill_To_Level" ("shared variable refnum in"), FALSE) -> (w277:bool)  [unwired: 1 in, 3 out]
        n163 = shared-variable-read(refnum<k21> "ni.var.psp://z004551/CDL0100 ReadWriteTags/HMI_ATank3_HeatEnable" ("shared variable refnum in"), FALSE) -> (w280:bool)  [unwired: 1 in, 3 out]
        n164 = local write "Drain Predip"(w288) -> ()
        n165 = local write "Drain"(w288) -> ()
        n166 = local write "Enable Auto Fill"(w277) -> ()
        n167 = local write "Enable Heat"(w280) -> ()
        n168 = shared-variable-read(refnum<k21> "ni.var.psp://z004551/CDL0100 ReadWriteTags/HMI_ATank3_Level_SetPnt" ("shared variable refnum in"), 0.0) -> (w274:dbl)  [unwired: 1 in, 3 out]
        n169 = local write "Enable Predip"(w297) -> ()
        n170 = shared-variable-read(refnum<k21> "ni.var.psp://z004551/CDL0100 ReadWriteTags/HMI_ATNK3_T_Setpoint" ("shared variable refnum in"), w285, 0.0) -> (w284:errorcluster, w283:dbl)  [unwired: 2 out]
        n171 = shared-variable-read(refnum<k21> "ni.var.psp://z004551/CDL0100 ReadWriteTags/HMI_Acid3_Tank_SG" ("shared variable refnum in"), 0.0) -> (w289:dbl)  [unwired: 1 in, 3 out]
        n172 = shared-variable-read(refnum<k21> "ni.var.psp://z004551/CDL0100 ReadWriteTags/HMI_Acid_Amount_PreDip" ("shared variable refnum in"), 0.0) -> (w271:dbl)  [unwired: 1 in, 3 out]
        n173 = shared-variable-read(refnum<k21> "ni.var.psp://z004551/CDL0100 ReadWriteTags/HMI_Dose_Acid_PreDip" ("shared variable refnum in"), FALSE) -> (w268:bool)  [unwired: 1 in, 3 out]
        n174 = shared-variable-read(refnum<k21> "ni.var.psp://z004551/CDL0100 ReadWriteTags/HMI_ATNK3_Flow_Setpoint" ("shared variable refnum in"), 0.0) -> (w294:dbl)  [unwired: 1 in, 3 out]
        n175 = local write "Level Setpoint"(w274) -> ()
        n176 = local write "Temperature Setpoint"(w283) -> ()
        n177 = local write "Specific Gravity"(w289) -> ()
        n178 = local write "Flow Setpoint"(w294) -> ()
        n179 = local write "Trig Sulfuric Predip"(w268) -> ()
        n180 = local write "Sulfuric Proc 1"(w271) -> ()
      }
      frame "Exit" {
        # "Destroy message queue >> this will halt the UI event handler loop"
        # "Stop the VI\n>> Perform any cleanup tasks in this message case.\n>> Clear display before closing."
        n181 = call <vilib>:"Destroy Message Queue.vi"("message queue in"=w301, "error in"=w302) -> ("error out"=w300:errorcluster)  [unwired: 11 in, 2 out]
        n182 = local write "status"("" ("Status")) -> ()
      }
      frame "---------- Application Operations ----------" {
        # "Dummy case to add a seperator in the Case Structure menu"
      }
      frame "Write_Tag" {
        n183 = call-poly <vilib>:"Write Message.vi"("error in"=w308, "data"=w305, "name"="WriteTag", "connection info in"=w306) -> ("error out"=w307:errorcluster)  [unwired: 6 in, 1 out]
      }
      frame "DisplayLastHr" {
        n184 = call "Trace Variable 1 hour Popup.vi"("Tag"=w311) -> ()  [unwired: 11 in]
      }
    }
  }
  n185 = call-poly <vilib>:"Get Connection Reference.vi"("error in"=w4, "connection info in"=w5) -> ("error out"=w8:errorcluster, "connection ID out"=w7:refnum<k5>)  [unwired: 8 out]
  n186 = TCP Close Connection(connection ID=w7, error in (no error)=w8) -> (error out=w10:errorcluster)  [unwired: 2 out]
  n187 = call <vilib>:"Error to Warning.vi"("1st Error to Convert"=w9, "error in"=w10) -> ("warning out"=w6:errorcluster)  [unwired: 3 in, 10 out]
  n188 = call <vilib>:"Simple Error Handler.vi"("error in (no error)"=w6) -> ()  [unwired: 4 in, 5 out]
